vi "SEND.vi"(8 "errin":errorcluster, 10 "chaîne":string, 11 "visa in":refnum<visa-resource-name>) -> (0 "errout":errorcluster, 2 "read buffer":string, 3 "visa out":refnum<visa-resource-name>)   [LabVIEW 2020]
uses:
  <vilib>/Instr/_visa.llb/VISA Configure Serial Port (Instr).vi
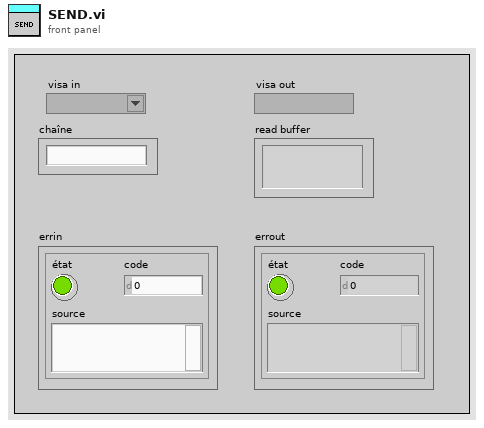
[diagram p1: front panel]
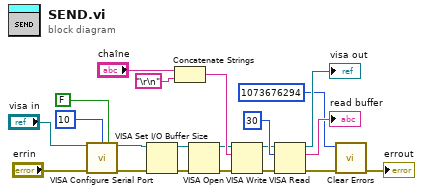
[diagram p0: block diagram]
diagram:
  n1 = call-poly "VISA Configure Serial Port"("VISA resource name"="visa in", "termination char\n(0xA = '\\n' = LF)"=u8 10 ("termination char\n(0xA = '\\n' = LF)"), "Enable Termination\nChar (T)"=FALSE ("Enable Termination\nChar (T)"), "error in (no error)"="errin") -> ("VISA resource name out"=w10:refnum<visa-resource-name>, "error out"=w5:errorcluster)  [unwired: 10 in]
  n2 = VISA Set I/O Buffer Size(VISA resource name=w10, error in (no error)=w5) -> (VISA resource name out=w11:refnum<visa-resource-name>, error out=w6:errorcluster)  [unwired: 2 in]
  n3 = Concatenate Strings("chaîne", "\r\n") -> (w16:string)
  n4 = VISA Open(error in (no error)=w6, VISA resource name=w11) -> (VISA resource name=w12:refnum<visa-resource-name>, error out=w7:errorcluster)  [unwired: 3 in]
  n5 = VISA Write(VISA resource name=w12, write buffer=w16, error in (no error)=w7) -> (VISA resource name out=w13:refnum<visa-resource-name>, error out=w8:errorcluster)  [unwired: 1 out]
  n6 = VISA Read(VISA resource name=w13, byte count=u32 30 ("nombre d'octets"), error in (no error)=w8) -> (VISA resource name out=→"visa out":refnum<visa-resource-name>, read buffer=→"read buffer":string, error out=w3:errorcluster)  [unwired: 1 out]
  n7 = call <vilib>:"Clear Errors.vi"("error in (no error)"=w3, "specific error code to clear (0: all)"=1073676294) -> ("error out"=→"errout":errorcluster)  [unwired: 4 in, 1 out]
